vi "DisplayLogic_DrawPlayfield.vi"(0 "Player":u8, 1 "ActivePixel":cluster{"h_pixel":i16, "v_pixel":i16}, 4 "PlayfieldPosition":T1) -> (15 "PixelData":bool[](array[boolean]), 18 "Draw":bool)   [LabVIEW 2018]
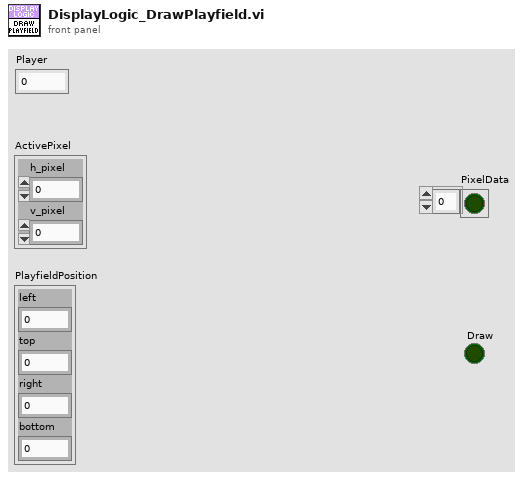
[diagram p1: front panel]
types:
  T1 = cluster{"left":i16, "top":i16, "right":i16, "bottom":i16}
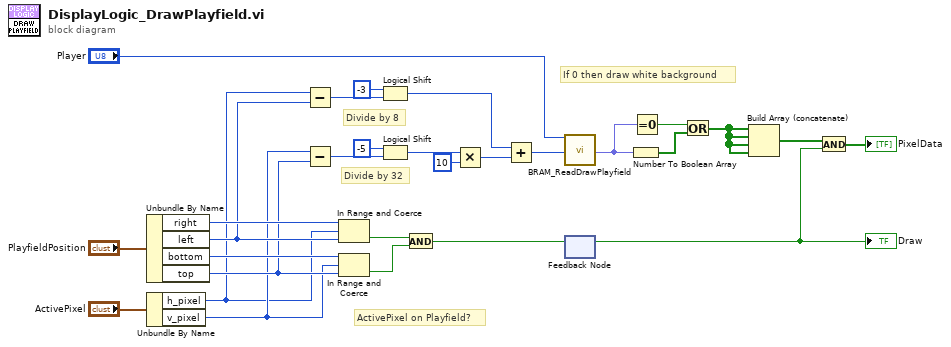
[diagram p0: block diagram]
diagram:
  # "If 0 then draw white background"
  # "Divide by 8"
  # "Divide by 32"
  # "ActivePixel on Playfield?"
  n1 = Unbundle By Name("PlayfieldPosition") -> ("right"=w28:i16, "left"=w27:i16, "bottom"=w26:i16, "top"=w4:i16)
  n2 = Unbundle By Name("ActivePixel") -> ("h_pixel"=w2:i16, "v_pixel"=w3:i16)
  n3 = Subtract(x=w2, y=w27) -> (x-y=w15:i16)
  n4 = Subtract(x=w3, y=w4) -> (x-y=w14:i16)
  n5 = In Range and Coerce(upper limit=w28, x=w2, lower limit=w27) -> (In Range?=w25:bool)  [unwired: 1 out]
  n6 = In Range and Coerce(upper limit=w26, x=w3, lower limit=w4) -> (In Range?=w24:bool)  [unwired: 1 out]
  n7 = Logical Shift(y=i16 -3, x=w15) -> (x << y=w20:i16)
  n8 = Logical Shift(y=i16 -5, x=w14) -> (x << y=w13:i16)
  n9 = And(x=w25, y=w24) -> (x .and. y?=w16:bool)
  n10 = Multiply(x=w13, y=i16 10) -> (x*y=w19:i16)
  n11 = Add(x=w20, y=w19) -> (x+y=w5:i16)
  n12 = call "BRAM_ReadDrawPlayfield.vi"("Player IN"="Player", "Address"=w5) -> ("Data"=w12:fxp<+,3,3>)  [unwired: 16 in, 1 out]
  n13 = feedback #1() -> (w7:bool)  [unwired: 1 in]
  "Draw" <- w7
  n14 = feedback-in #1(w16) -> ()
  n15 = Number To Boolean Array(number=w12) -> (Boolean array=w10:bool[])
  n16 = Equal To 0?(x=w12) -> (x = 0?=w11:bool)
  n17 = Or(x=w11, y=w10) -> (x .or. y?=w1:bool[])
  n18 = Build Array (concatenate)(w1, w1, w1, w1) -> (w8:bool[])
  n19 = And(x=w8, y=w7) -> (x .and. y?=→"PixelData":bool[])
